vi "TCP Engine AIO&DIO JSON Conversion.vi"(8 "error in":errorcluster, 10 "Interface":string, 11 "JSON String":string) -> (0 "error out":errorcluster, 1 "Data":variant, 2 "SubCmd":string, 3 "Command":string)   [LabVIEW 2018, in "TCP Engine.lvlib"]
doc: "All Rights Reserved © 2017 SyncSols"
uses:
  TCP Engine.lvlib
  Controls/JSON Analog Start&Update.ctl
  Controls/JSON Analog Configure.ctl
  Controls/JSON Digital Start&Update.ctl
  Controls/JSON Digital Configure.ctl
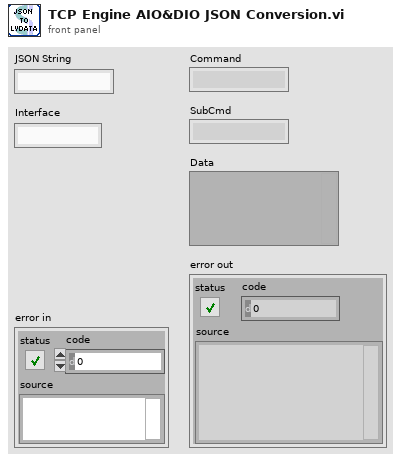
[diagram p1: front panel]
types:
  T1 = typedef "TCP Engine.lvlib/JSON Analog Configure.ctl" = cluster{"Command":string, "SubCmd":string, "Data":cluster{"Channel":string, "Min Voltage":dbl, "Max Voltage":dbl}[]}
  T2 = typedef "TCP Engine.lvlib/JSON Analog Start&Update.ctl" = cluster{"Command":string, "SubCmd":string, "Data":i32[]}
  T3 = typedef "TCP Engine.lvlib/JSON Digital Configure.ctl" = cluster{"Command":string, "SubCmd":string, "Data":string[]}
  T4 = typedef "TCP Engine.lvlib/JSON Digital Start&Update.ctl" = cluster{"Command":string, "SubCmd":string, "Data":i32[]}
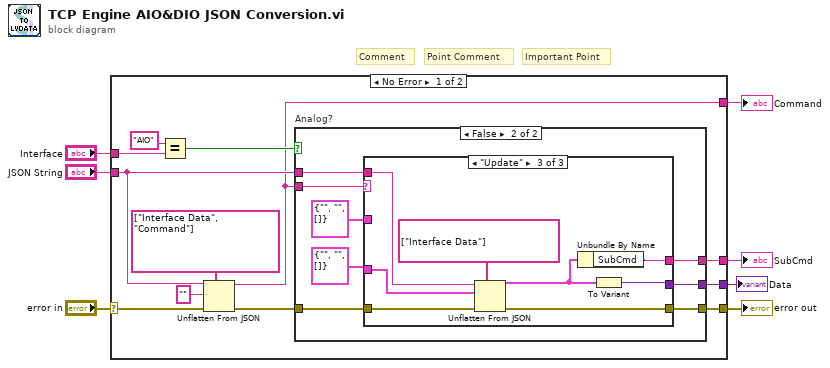
[diagram p0: block diagram]
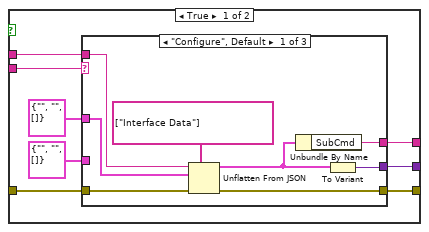
[diagram p2: hidden frame]
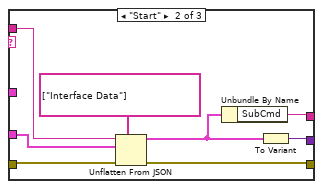
[diagram p3: hidden frame]
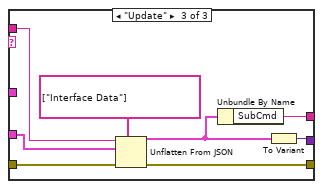
[diagram p4: hidden frame]
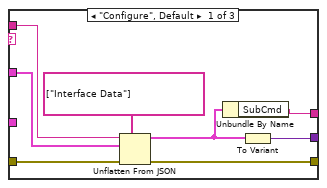
[diagram p5: hidden frame]
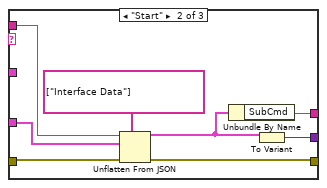
[diagram p6: hidden frame]
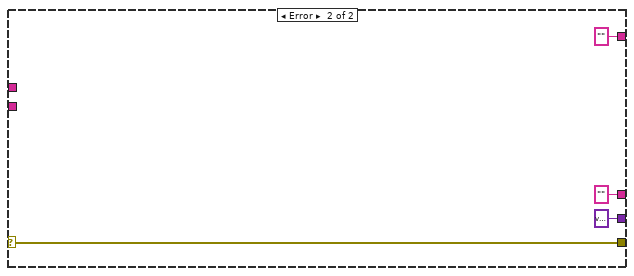
[diagram p7: hidden frame]
diagram:
  # "Important Point"
  # "Point Comment"
  # "Comment"
  n1 = case shown="No Error" "error in" {
    selector: "error in" -> [w19 w87]
    tunnel: [w14 w87] -> w7
    tunnel: "JSON String" -> [w16 _]
    tunnel: "Interface" -> [w12 _]
    tunnel: [w10 "" ("SubCmd")] -> w3
    tunnel: [w9 ""] -> w2
    tunnel: [w8 variant ("Variant")] -> w1
    frame No Error {
      n2 = Equal?(x="AIO", y=w12) -> (x = y?=w13:bool)
      n3 = Unflatten From JSON(path=string[] ["Interface Data", "Command"], JSON string=w16, type and defaults="", error in (no error)=w19) -> (value=w9:string, error out=w15:errorcluster)  [unwired: 3 in]
      n4 = case "Analog?" shown="False" w13 {
        tunnel: w9 -> [w27 w59]
        tunnel: w16 -> [w25 w58]
        tunnel: w15 -> [w23 w56]
        tunnel: [w22 w55] -> w14
        tunnel: [w21 w53] -> w10
        tunnel: [w20 w52] -> w8
        frame True {
          n5 = case shown="\"Configure\", Default" w27 {
            tunnel: T1 {"Command"="", "SubCmd"="", "Data"=[]} -> [w34 _ _]
            tunnel: w25 -> [w33 w42 w50]
            tunnel: T2 {"Command"="", "SubCmd"="", "Data"=[]} -> [_ w41 w46]
            tunnel: w23 -> [w32 w40 w49]
            tunnel: [w31 w39 w48] -> w22
            tunnel: [w30 w38 w47] -> w20
            tunnel: [w28 w36 w44] -> w21
            frame "Configure", Default {
              n6 = Unflatten From JSON(path=string[] ["Interface Data"], JSON string=w33, type and defaults=w34, error in (no error)=w32) -> (value=w29:T1, error out=w31:errorcluster)  [unwired: 3 in]
              n7 = Unbundle By Name(w29) -> ("SubCmd"=w28:string)
              n8 = To Variant(anything=w29) -> (Variant=w30:variant)
            }
            frame "Start" {
              n9 = Unflatten From JSON(path=string[] ["Interface Data"], JSON string=w42, type and defaults=w41, error in (no error)=w40) -> (value=w37:T2, error out=w39:errorcluster)  [unwired: 3 in]
              n10 = Unbundle By Name(w37) -> ("SubCmd"=w36:string)
              n11 = To Variant(anything=w37) -> (Variant=w38:variant)
            }
            frame "Update" {
              n12 = Unflatten From JSON(path=string[] ["Interface Data"], JSON string=w50, type and defaults=w46, error in (no error)=w49) -> (value=w45:T2, error out=w48:errorcluster)  [unwired: 3 in]
              n13 = Unbundle By Name(w45) -> ("SubCmd"=w44:string)
              n14 = To Variant(anything=w45) -> (Variant=w47:variant)
            }
          }
        }
        frame False {
          n15 = case shown="\"Update\"" w59 {
            tunnel: T3 {"Command"="", "SubCmd"="", "Data"=[]} -> [w66 _ _]
            tunnel: w58 -> [w65 w74 w82]
            tunnel: T4 {"Command"="", "SubCmd"="", "Data"=[]} -> [_ w73 w78]
            tunnel: w56 -> [w64 w72 w81]
            tunnel: [w63 w71 w80] -> w55
            tunnel: [w62 w70 w79] -> w52
            tunnel: [w60 w68 w76] -> w53
            frame "Configure", Default {
              n16 = Unflatten From JSON(path=string[] ["Interface Data"], JSON string=w65, type and defaults=w66, error in (no error)=w64) -> (value=w61:T3, error out=w63:errorcluster)  [unwired: 3 in]
              n17 = Unbundle By Name(w61) -> ("SubCmd"=w60:string)
              n18 = To Variant(anything=w61) -> (Variant=w62:variant)
            }
            frame "Start" {
              n19 = Unflatten From JSON(path=string[] ["Interface Data"], JSON string=w74, type and defaults=w73, error in (no error)=w72) -> (value=w69:T4, error out=w71:errorcluster)  [unwired: 3 in]
              n20 = Unbundle By Name(w69) -> ("SubCmd"=w68:string)
              n21 = To Variant(anything=w69) -> (Variant=w70:variant)
            }
            frame "Update" {
              n22 = Unflatten From JSON(path=string[] ["Interface Data"], JSON string=w82, type and defaults=w78, error in (no error)=w81) -> (value=w77:T4, error out=w80:errorcluster)  [unwired: 3 in]
              n23 = Unbundle By Name(w77) -> ("SubCmd"=w76:string)
              n24 = To Variant(anything=w77) -> (Variant=w79:variant)
            }
          }
        }
      }
    }
    frame Error {
    }
  }
  "error out" <- w7
  "SubCmd" <- w3
  "Command" <- w2
  "Data" <- w1
